vi "Points to Oval.vi"(8 "Size":dbl, 10 "Point Array":T1[](array[typedef]) {"Y" format="%.2f"; "X" format="%.2f"}, 11 "Image In":T2) -> (3 "Image Out":T2(plugin-control))   [LabVIEW 2022 SP3]
uses:
  <vilib>/vision/Image Controls.llb/IMAQ Image.ctl
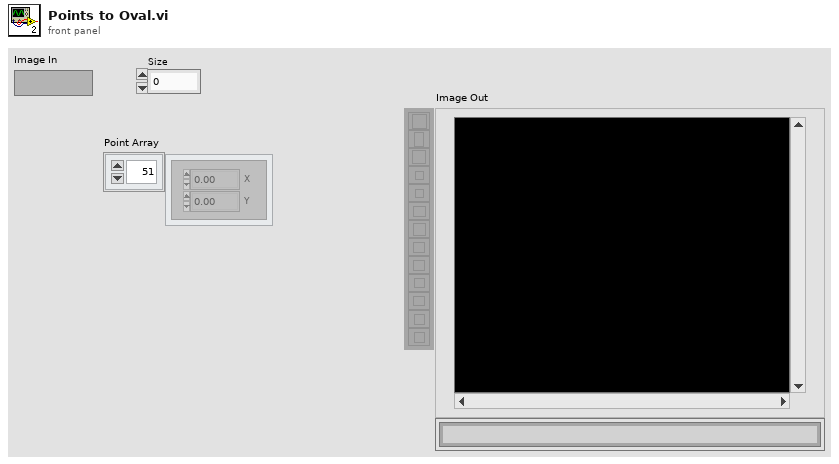
[diagram p1: front panel]
types:
  T1 = typedef "IMAQ Point" = cluster{"X":sgl, "Y":sgl}
  T2 = typedef "IMAQ Image.ctl" = refnum<image>
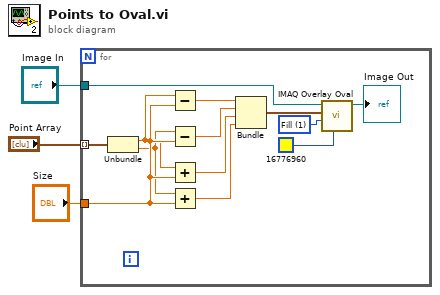
[diagram p0: block diagram]
diagram:
  n1 = for {
    tunnel: "Size" -> [w12]
    tunnel: "Image In" -> [w9]
    tunnel: "Point Array" -> [w6] mode=indexing
    w7 = u32 1 items=["Frame", "Fill"] ("Drawing Mode (Frame)")
    n2 = Unbundle(w6) -> ("X"=w5:sgl, "Y"=w4:sgl)
    n3 = Subtract(x=w5, y=w12) -> (x-y=w16:dbl)
    n4 = Subtract(x=w4, y=w12) -> (x-y=w15:dbl)
    n5 = Add(x=w5, y=w12) -> (x+y=w14:dbl)
    n6 = Add(x=w4, y=w12) -> (x+y=w13:dbl)
    n7 = Bundle(w16, w15, w14, w13) -> (w11:cluster{dbl, dbl, dbl, dbl})  [unwired: 1 in]
    n8 = call "IMAQ Overlay Oval"("Color"=u32 16776960, "Drawing Mode (Frame)"=w7, "Bounding Rectangle"=w11, "Image"=w9) -> ("Image Out"=→"Image Out":T2)  [unwired: 6 in, 1 out]
  }
